vi "get table and column names.vi"() -> ()   [LabVIEW 2020]
uses:
  Database OOP/Database Libraries/ADODB/ADODB Class/ADODB.lvclass
  Database OOP/Database Libraries/ADODB/UDL Connection Class/UDL Connection.lvclass
  C:/Users/User/Desktop/Raman Program/Database OOP/source/Database OOP/Database Libraries/Database Interfaces/Database Connection Class/Database Connection.lvclass
panel:
  in  "Database *.udl file":path=path "C:/Users/User/Desktop/Raman Program/Test Data/testDB.udl"
  out "Table and Column Info":T1(array[cluster])
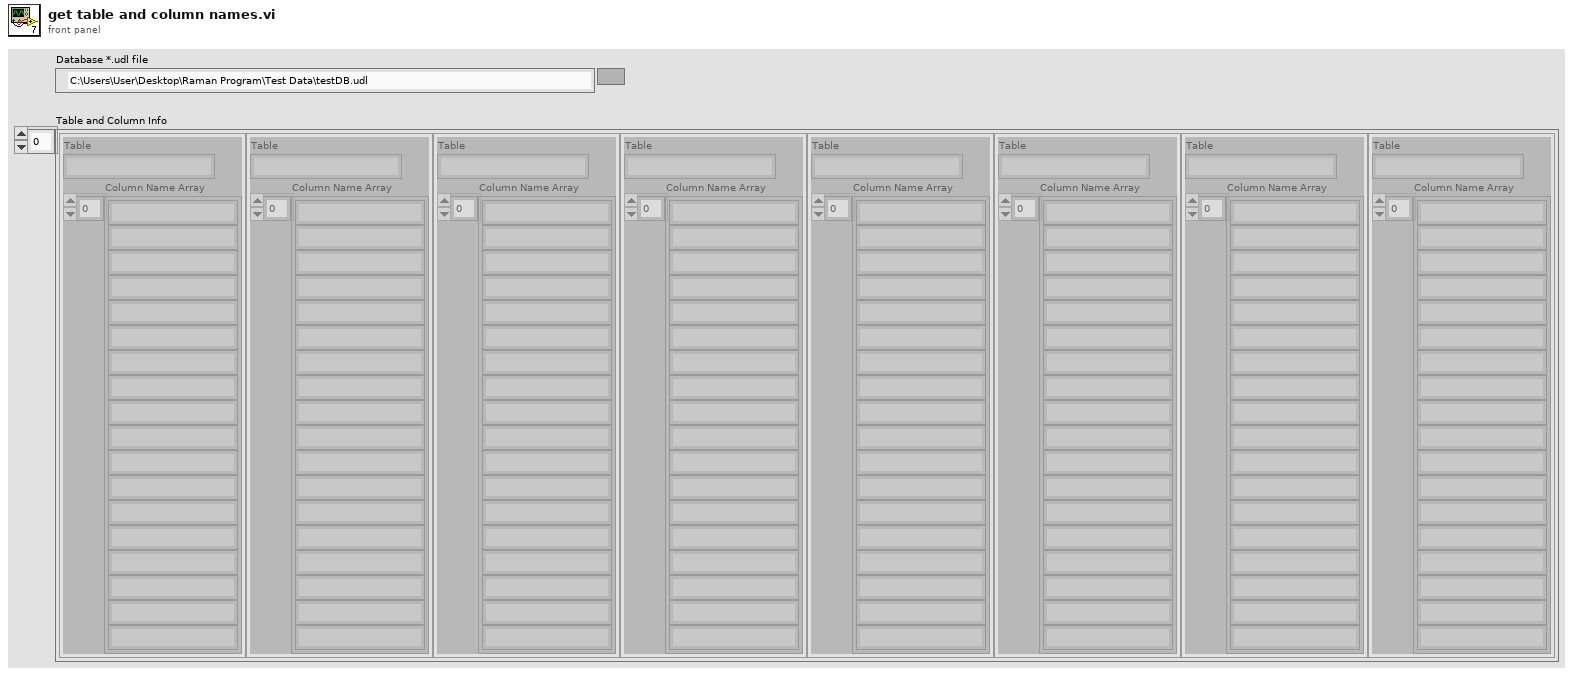
[diagram p1: front panel]
types:
  T1 = cluster{"Table":string, "Column Name Array":string[]}[]
  T2 = cluster{"Table":string, "Column Name Array":string[]}
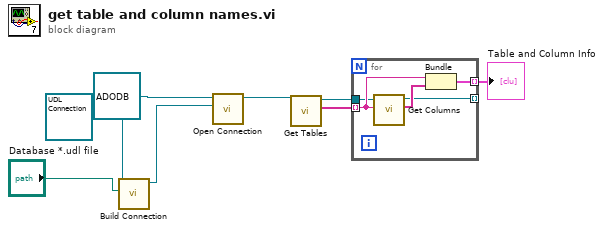
[diagram p0: block diagram]
diagram:
  n1 = call "Build Connection.vi"("*.udl file path"="Database *.udl file", "UDL Connection in"=refnum<class "UDL Connection.lvclass"> refnum) -> ("UDL Connection out"=w2:refnum<class "UDL Connection.lvclass">)  [unwired: 8 in, 1 out]
  n2 = call-dynamic "Open Connection.vi"("Connection"=w2, "ADODB in"=refnum<class "ADODB.lvclass"> refnum ("ADODB.lvlib:ADODB.lvclass")) -> ("ADODB out"=w7:refnum<class "ADODB.lvclass">)  [unwired: 8 in, 1 out]
  n3 = call-dynamic "Get Tables.vi"("ODBC in"=w7) -> ("Table Names"=w8:string[], "ODBC out"=w6:refnum<class "ADODB.lvclass">)  [unwired: 8 in, 1 out]
  n4 = for {
    tunnel: w8 -> [w12] mode=indexing
    tunnel: [w11] -> w5 mode=indexing
    tunnel: w6 -> [w10]
    tunnel: [w9] -> _ mode=indexing
    n5 = call-dynamic "Get Columns.vi"("Table Name"=w12, "ADODB in"=w10) -> ("Column Name Array"=w13:string[], "ADODB out"=w9:refnum<class "ADODB.lvclass">)  [unwired: 7 in, 1 out]
    n6 = Bundle("Table"=w12, "Column Name Array"=w13) -> (w11:T2)  [unwired: 1 in]
  }
  "Table and Column Info" <- w5
